vi "LIA_DAQ_Read.vi"(8 "error in (no error)":errorcluster, 10 "Subscribe Path Array":string[](array[string]), 11 "DAQ ModHandle In":T1 {"ModHandle" format="0x%08x"; "Conn" format="0x%08x"}) -> (0 "error out":errorcluster, 2 "Grid DEMOD R":dbl[][](array[numeric]), 3 "DAQ ModHandle Out":T1 {"ModHandle" format="0x%08x"; "Conn" format="0x%08x"})   [LabVIEW 2016, in "ZI LIA.lvlib"]
uses:
  ZI LIA.lvlib
  <instrlib>/Zurich Instruments LabOne/Public/Modules/ziTypeModHandle.ctl
  <instrlib>/Zurich Instruments LabOne/Public/Modules/ziModGetDoubleData.vi
  <instrlib>/Zurich Instruments LabOne/Zurich Instruments LabOne.lvlib
panel:
  out "Finished?":bool
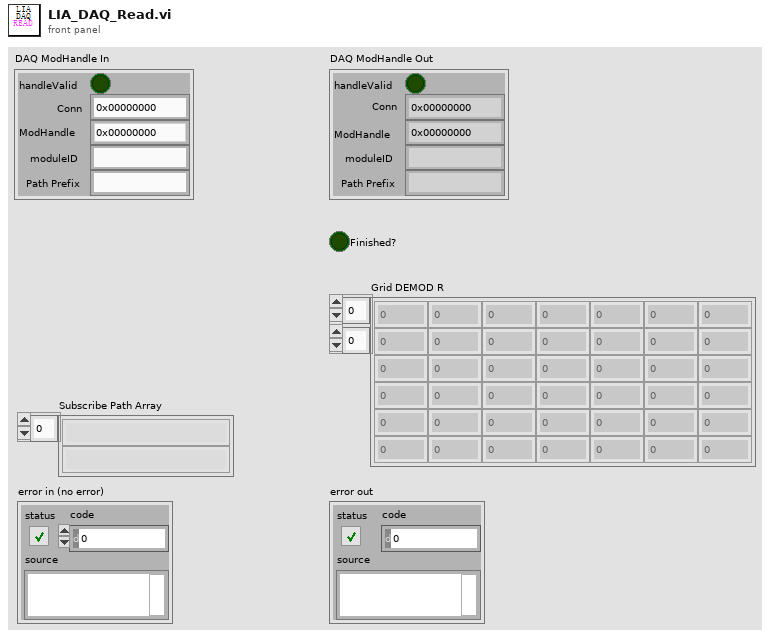
[diagram p1: front panel]
types:
  T1 = typedef "Zurich Instruments LabOne.lvlib/ziTypeModHandle.ctl" = cluster{"handleValid":bool, "Conn":u64, "ModHandle":u64, "moduleID":string, "Path Prefix":string}
  T2 = typedef "Zurich Instruments LabOne.lvlib/ziTypeModResults.ctl" = cluster{"PathArray":string[], "ValueType":T3, "NoOfResults":u64, "ziGenericHeader":T4[]}
  T3 = typedef "Zurich Instruments LabOne.lvlib/ziTypePollType.ctl" = enum16{"NONE", "DOUBLE_DATA", "INTEGER_DATA", "DEMOD_SAMPLE", "SCOPE_WAVE_HF2", "AUXIN_SAMPLE", "DIO_SAMPLE", "BYTE_ARRAY", "PWA_WAVE", "9", "10", "11", "12", "13", "14", "15", "TREE_CHANGE_DEPRI", "17", "ERROR", "19", "20", "21", "22", "23", "24", "25", "26", "27", "28", "29", "30", "31", "DOUBLE_DATA_TS", "INTEGER_DATA_TS", "34", "SCOPE_WAVE", "SCOPE_WAVE_EX", "37", "BYTE_ARRAY_TS", "39", "40", "41", "42", "43", "44", "45", "CNT_DATA", "47", "TREE_CHANGE", "49", "50", "51", "52", "53", "54", "55", "56", "57", "58", "59", "60", "61", "62", "63", "SWEEPER_DATA", "SPECTRUM_DATA", "ADVISOR_DATA", "VECTOR_DATA", "IMP_DATA"}
  T4 = typedef "Zurich Instruments LabOne.lvlib/ziTypeModGenericHeader.ctl" = cluster{"HeaderType":enum8{"HEADER_TYPE_NONE", "HEADER_TYPE_SWTRIGGER", "HEADER_TYPE_SWEEPER"}, "SampleFormat":u8, "SystemTime":timestamp, "CreatedTimeStamp":u64, "ChangedTimeStamp":u64, "Flags":u32, "ChunkSizeBytes":u64, "Name":string, "Status":u32, "GroupIndex":u32, "Color":u32, "ActiveRow":u32, "TriggerNumber":u64, "GridRows":u32, "GridCols":u32, "GridMode":u32, "GridOperation":u32, "GridDirection":u32, "GridRepetitions":u32, "GridColDelta":dbl, "GridColOffset":dbl, "GridRowDelta":dbl, "GridRowOffset":dbl, "Bandwidth":dbl, "Center":dbl, "Nenbw":dbl}
  T5 = typedef "Zurich Instruments LabOne.lvlib/ziTypeDoubleDataTSGrid.ctl" = cluster{"Timestamp (ticks)":u64[][], "Value":dbl[][]}
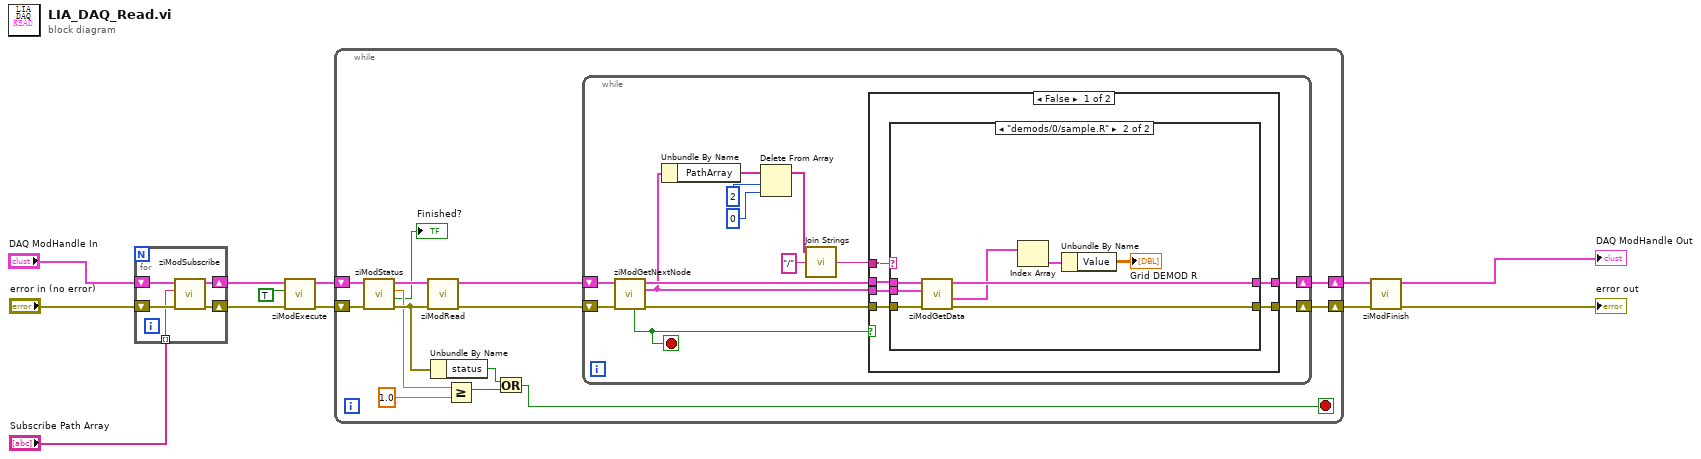
[diagram p0: block diagram]
diagram:
  n1 = for {
    tunnel: "Subscribe Path Array" -> [w13] mode=indexing
    shift-right: [w17] -> w5
    shift-left: "DAQ ModHandle In" -> [w15]
    shift-right: [w16] -> w6
    shift-left: "error in (no error)" -> [w14]
    n2 = call <instrlib>:"ziModSubscribe.vi"("Error In"=w14, "Path"=w13, "ModHandle In"=w15) -> ("Error Out"=w16:errorcluster, "ModHandle Out"=w17:T1)  [unwired: 6 in]
  }
  n3 = call <instrlib>:"ziModExecute.vi"("Error In"=w6, "Modal (F)"=TRUE, "ziModHandle In"=w5) -> ("Error Out"=w12:errorcluster, "ziModHandle Out"=w11:T1)  [unwired: 5 in, 1 out]
  n4 = while {
    shift-right: [w30] -> w4
    shift-left: w11 -> [w25]
    shift-right: [w31] -> w3
    shift-left: w12 -> [w24]
    stop <- w18 stop-if-true
    n5 = call <instrlib>:"ziModStatus.vi"("Error In"=w24, "ModHandle IN"=w25) -> ("Error Out"=w26:errorcluster, "Finished?"=→"Finished?":bool, "Progress (unity)"=w23:dbl, "ModHandle Out"=w27:T1)  [unwired: 5 in]
    n6 = call <instrlib>:"ziModRead.vi"("error in"=w26, "ziModHandle In"=w27) -> ("error out"=w29:errorcluster, "ziModHandle Out"=w28:T1)  [unwired: 8 in]
    n7 = Unbundle By Name(w26) -> ("status"=w20:bool)
    n8 = Greater Or Equal?(x=w23, y=1.0) -> (x >= y?=w21:bool)
    n9 = Or(x=w20, y=w21) -> (x .or. y?=w18:bool)
    n10 = while {
      shift-right: [w40] -> w30
      shift-left: w28 -> [w44]
      shift-right: [w41] -> w31
      shift-left: w29 -> [w45]
      stop <- w39 stop-if-true
      n11 = call <instrlib>:"ziModGetNextNode.vi"("Error In"=w45, "ModHandle In"=w44) -> ("Error Out"=w42:errorcluster, "ModResults"=w38:T2, "ModHandle Out"=w43:T1, "NoData"=w39:bool)  [unwired: 6 in]
      n12 = Unbundle By Name(w38) -> ("PathArray"=w37:string[])
      n13 = Delete From Array(array=w37, length=2, index=0) -> (array with subset deleted=w34:string[])  [unwired: 1 out]
      n14 = call <vilib>:"Join Strings.vi"("Separator (,)"="/", "Strings In"=w34) -> ("String"=w32:string)  [unwired: 1 in]
      n15 = case shown="False" w39 {
        tunnel: w38 -> [w51 _]
        tunnel: w43 -> [w50 w63]
        tunnel: w42 -> [w49 w62]
        tunnel: [w48 w62] -> w41
        tunnel: [w47 w63] -> w40
        tunnel: w32 -> [w46 _]
        frame False {
          n16 = case shown="\"demods/0/sample.R\"" w46 {
            tunnel: w50 -> [w53 w56]
            tunnel: w51 -> [_ w55]
            tunnel: w49 -> [w52 w59]
            tunnel: [w52 w60] -> w48
            tunnel: [w53 w61] -> w47
            frame Default {
            }
            frame "demods/0/sample.R" {
              n17 = call-poly <instrlib>:"ziModGetData.vi"("Error In"=w59, "ModResults"=w55, "ModHandle In"=w56) -> ("Error Out"=w60:errorcluster, "DoubleSampleGrid"=w58:T5[], "ModHandle Out"=w61:T1)  [unwired: 4 in, 2 out]
              n18 = Index Array(array=w58) -> (element=w57:T5)  [unwired: 1 in]
              n19 = Unbundle By Name(w57) -> ("Value"=→"Grid DEMOD R":dbl[][])
            }
          }
        }
        frame True {
        }
      }
    }
  }
  n20 = call <instrlib>:"ziModFinish.vi"("Error In"=w3, "ziModHandle In"=w4) -> ("Error Out"=→"error out":errorcluster, "ziModHandle Out"=→"DAQ ModHandle Out":T1)  [unwired: 7 in]
